vi "Get Foreground Window.vi"(8 "error in":errorcluster {"code" format="%d\n%x"}) -> (0 "error out":errorcluster {"code" format="%d\n%x"}, 2 "window name":string, 3 "window refnum out":T1)   [LabVIEW 2020, in "MacroAssert.lvlib" / "Win Util.lvlib"]
doc: "Gets the refnum of the frontmost (foreground) window."
uses:
  Win Util.lvlib
  user32.dll
  Window Refnum.ctl
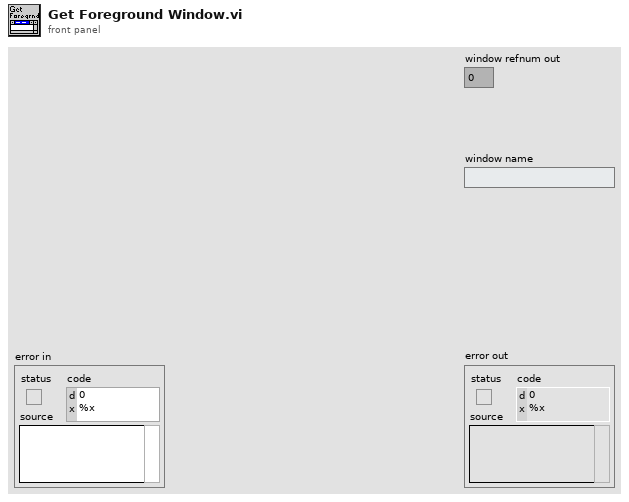
[diagram p1: front panel]
types:
  T1 = typedef "MacroAssert.lvlib/Win Util.lvlib/Window Refnum.ctl" = u64
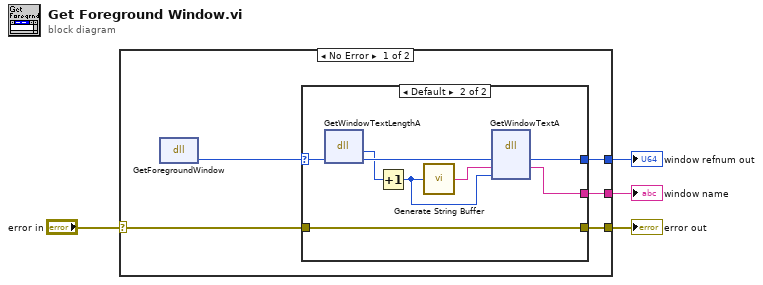
[diagram p0: block diagram]
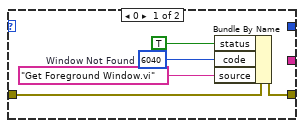
[diagram p2: hidden frame]
diagram:
  n1 = case shown="No Error" "error in" {
    selector: "error in" -> [w9 w23]
    tunnel: [w8 w23] -> w3
    tunnel: [w6 _] -> w4
    tunnel: [w5 _] -> w2
    frame No Error {
      n2 = dll-call lib="user32.dll" fn="GetForegroundWindow"() -> ("hWnd"=w7:u64)  [unwired: 3 in, 2 out]
      n3 = case shown="Default" w7 {
        selector: w7 -> [_ w15]
        tunnel: w9 -> [w11 w20]
        tunnel: [w14 w20] -> w8
        tunnel: [_ w19] -> w6
        tunnel: [_ w18] -> w5
        frame 0 {
          w13 = 6040  # Window Not Found
          n4 = Bundle By Name(cluster=w11, "status"=TRUE ("show call chain? (False)"), "code"=w13, "source"="Get Foreground Window.vi") -> (w14:errorcluster)
        }
        frame Default {
          n5 = dll-call lib="user32.dll" fn="GetWindowTextLengthA" label="GetWindowTextLength"("hWnd"=w15) -> ("length"=w17:i32, "hWnd"=w21:u64)  [unwired: 3 in, 2 out]
          n6 = Increment(x=w17) -> (x+1=w16:i32)
          n7 = call "Generate String Buffer.vi"("buffer size"=w16) -> ("string buffer"=w22:string)
          n8 = dll-call lib="user32.dll" fn="GetWindowTextA" label="GetWindowText"("hWnd"=w21, "NameBuffer"=w22, "MaxCharsToCopy"=w16) -> ("hWnd"=w18:u64, "NameBuffer"=w19:string)  [unwired: 4 in, 3 out]
        }
      }
    }
    frame Error {
    }
  }
  "error out" <- w3
  "window name" <- w4
  "window refnum out" <- w2
